vi "Read Trigger Light Camera Sequence Opcode_MI.vi"(8 "error in (no error)":errorcluster, 9 "Status":string, 10 "Light Sequence Trigger":string, 11 "MachineInterfaceRecipeOpcodes":T1) -> (0 "error out":errorcluster, 3 "Trigger Light Camera Sequence Opcode":string[](array[string]))   [LabVIEW 2019, in "Machine Interface.lvclass"]
uses:
  Machine Interface.lvclass
  Controls/Machine Interface Config File Structure_MI.ctl
panel:
  out "Path list":string[](array[string])
  out "Error Message":string
  out "VCluster\n out":variant
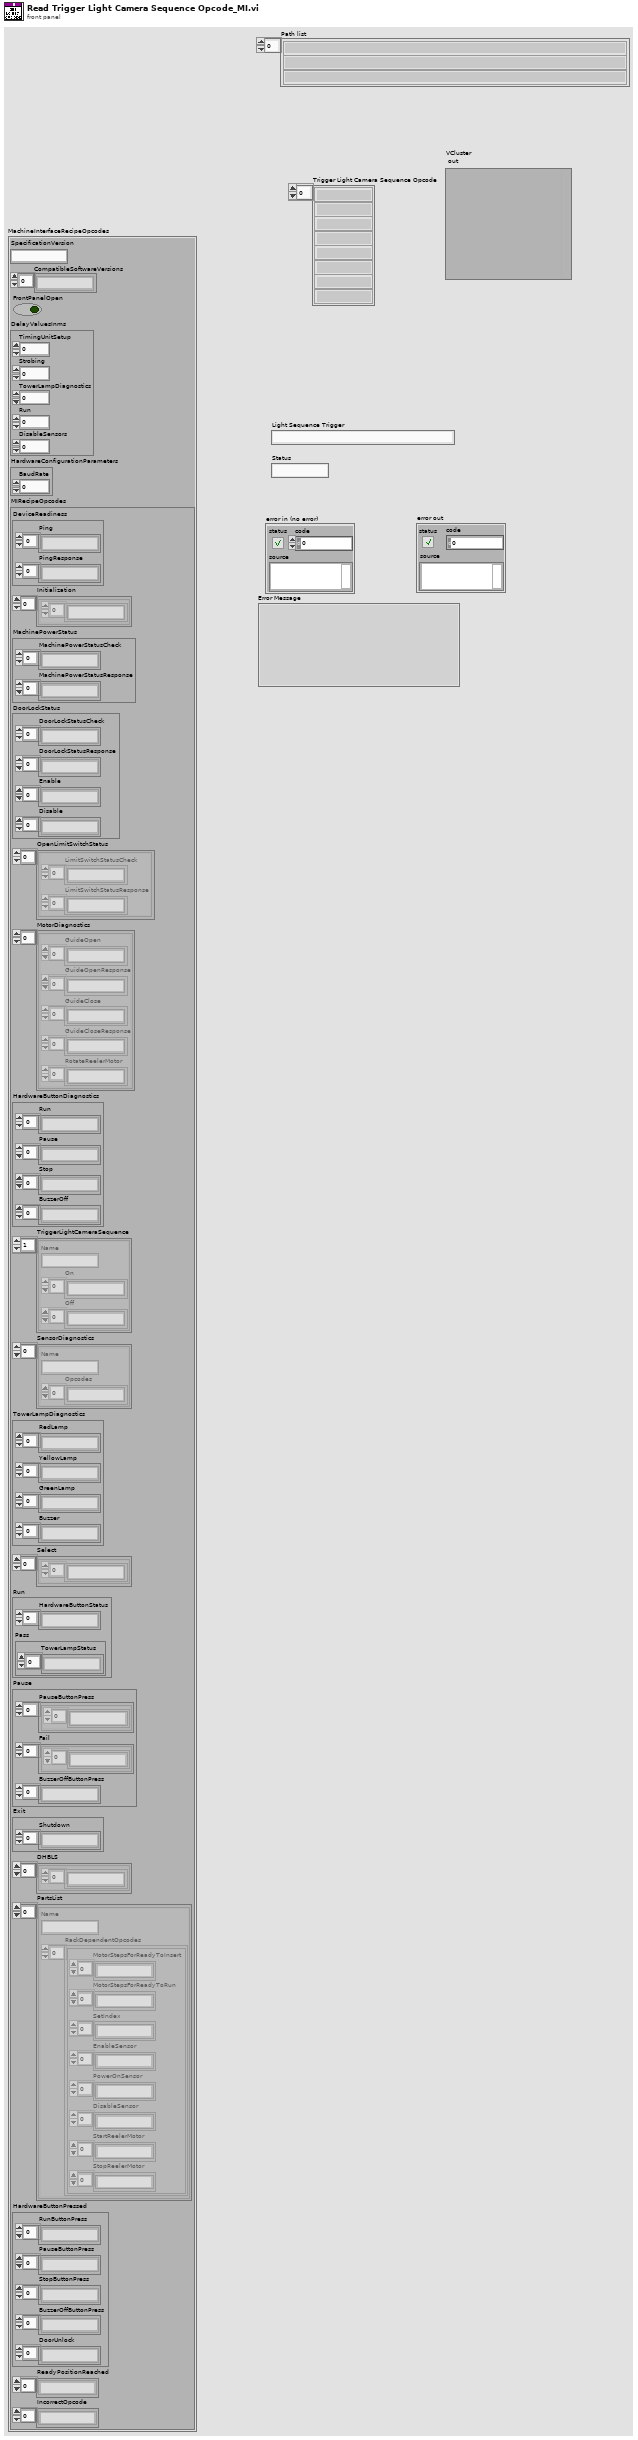
[diagram p1: front panel]
types:
  T1 = typedef "Machine Interface.lvclass/Machine Interface Config File Structure_MI.ctl" = cluster{"SpecificationVersion":string, "CompatibleSoftwareVersions":string[], "FrontPanelOpen":bool, "DelayValuesInms":cluster{"TimingUnitSetup":i32, "Strobing":i32, "TowerLampDiagnostics":i32, "Run":i32, "DisableSensors":i32}, "HardwareConfigurationParameters":cluster{"BaudRate":dbl}, "MIRecipeOpcodes":cluster{"DeviceReadiness":cluster{"Ping":string[], "PingResponse":string[]}, "Initialization":cluster{string[]}[], "MachinePowerStatus":cluster{"MachinePowerStatusCheck":string[], "MachinePowerStatusResponse":string[]}, "DoorLockStatus":cluster{"DoorLockStatusCheck":string[], "DoorLockStatusResponse":string[], "Enable":string[], "Disable":string[]}, "OpenLimitSwitchStatus":cluster{"LimitSwitchStatusCheck":string[], "LimitSwitchStatusResponse":string[]}[], "MotorDiagnostics":cluster{"GuideOpen":string[], "GuideOpenResponse":string[], "GuideClose":string[], "GuideCloseResponse":string[], "RotateReelerMotor":string[]}[], "HardwareButtonDiagnostics":cluster{"Run":string[], "Pause":string[], "Stop":string[], "BuzzerOff":string[]}, "TriggerLightCameraSequence":cluster{"Name":string, "On":string[], "Off":string[]}[], "SensorDiagnostics":cluster{"Name":string, "Opcodes":string[]}[], "TowerLampDiagnostics":cluster{"RedLamp":string[], "YellowLamp":string[], "GreenLamp":string[], "Buzzer":string[]}, "Select":cluster{string[]}[], "Run":cluster{"HardwareButtonStatus":string[], "Pass":cluster{"TowerLampStatus":string[]}}, "Pause":cluster{"PauseButtonPress":cluster{string[]}[], "Fail":cluster{string[]}[], "BuzzerOffButtonPress":string[]}, "Exit":cluster{"Shutdown":string[]}, "DHBLS":cluster{string[]}[], "PartsList":cluster{"Name":string, "RackDependentOpcodes":cluster{"MotorStepsForReadyToInsert":string[], "MotorStepsForReadyToRun":string[], "SetIndex":string[], "EnableSensor":string[], "PowerOnSensor":string[], "DisableSensor":string[], "StartReelerMotor":string[], "StopReelerMotor":string[]}[]}[], "HardwareButtonPressed":cluster{"RunButtonPress":string[], "PauseButtonPress":string[], "StopButtonPress":string[], "BuzzerOffButtonPress":string[], "DoorUnlock":string[]}, "ReadyPositionReached":string[], "IncorrectOpcode":string[]}}
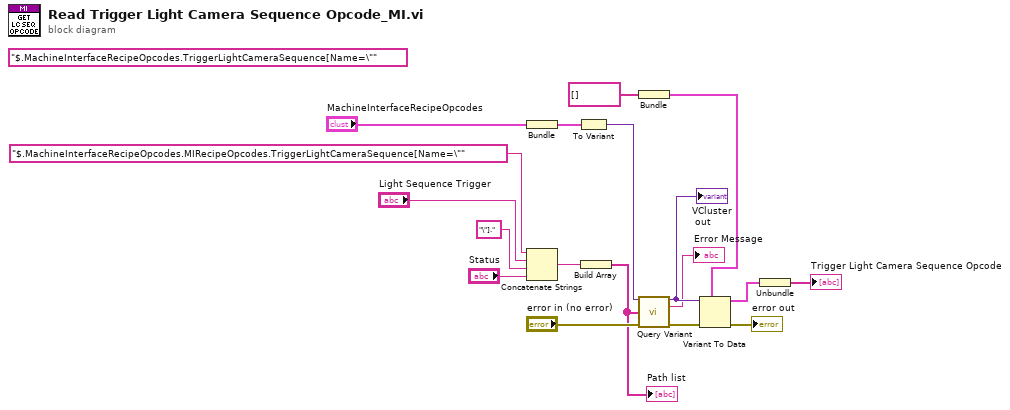
[diagram p0: block diagram]
diagram:
  (unwired) "$.MachineInterfaceRecipeOpcodes.TriggerLightCameraSequence[Name=\"" ("String")
  n1 = Bundle("MachineInterfaceRecipeOpcodes"="MachineInterfaceRecipeOpcodes") -> (w7:cluster{"MachineInterfaceRecipeOpcodes":T1})  [unwired: 1 in]
  n2 = Concatenate Strings("$.MachineInterfaceRecipeOpcodes.MIRecipeOpcodes.TriggerLightCameraSequence[Name=\"" ("String"), "Light Sequence Trigger", "\"]." ("string"), "Status") -> (w10:string)
  n3 = To Variant(anything=w7) -> (Variant=w4:variant)
  n4 = Build Array(w10) -> (w2:string[])
  "Path list" <- w2
  n5 = Bundle(string[] []) -> (w16:cluster{string[]})  [unwired: 1 in]
  n6 = call <vilib>:"Query Variant.vi"("VCluster in"=w4, "pathList"=w2, "error IO"="error in (no error)") -> ("VCluster\n out"=w3:variant, "Error Message"=→"Error Message":string, "error out"=w6:errorcluster)  [unwired: 9 in, 1 out]
  "VCluster\n out" <- w3
  n7 = Variant To Data(error in=w6, type=w16, Variant=w3) -> (data=w17:cluster{string[]}, error out=→"error out":errorcluster)
  n8 = Unbundle(w17) -> (→"Trigger Light Camera Sequence Opcode":string[])
